vi "test - Round Trip -Array of Cluster of Enum and Array - Cluster.vi"(8 "error in (no error)":errorcluster, 11 "TestCase in":refnum<class "Python Data Tools Tests.lvclass">) -> (0 "error out":errorcluster, 3 "TestCase out":refnum<class "Python Data Tools Tests.lvclass">)   [LabVIEW 2013, in "Python Data Tools Tests.lvclass"]
uses:
  Python Data Tools Tests.lvclass
  <vilib>/addons/_JKI Toolkits/VI Tester/TestCase.llb/TestCase.lvclass
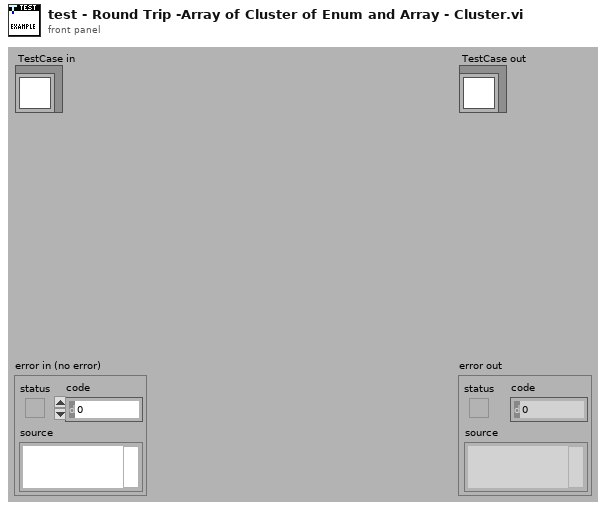
[diagram p1: front panel]
types:
  T1 = cluster{enum16{"Case1", "Case2", "AnotherCase"}, i32[]}[]
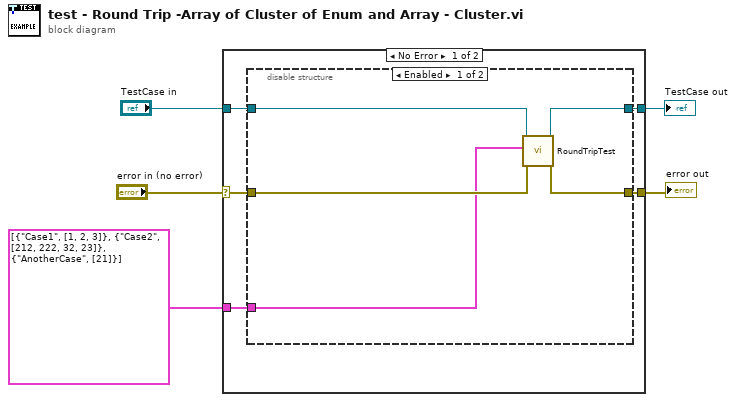
[diagram p0: block diagram]
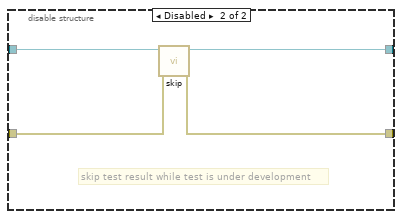
[diagram p2: hidden frame]
diagram:
  n1 = case shown="No Error" "error in (no error)" {
    selector: "error in (no error)" -> [w8 w21]
    tunnel: [w7 w21] -> w4
    tunnel: [w9 w20] -> w2
    tunnel: "TestCase in" -> [w10 w20]
    tunnel: T1 [{enum."Case1", [1, 2, 3]}, {enum."Case2", [212, 222, 32, 23]}, {enum."AnotherCase", [21]}] -> [w6 _]
    frame No Error {
      n2 = disable-structure shown="Enabled" {
        disable-tunnel: w10 -> [w15 w19]
        disable-tunnel: [w14 w16] -> w9
        disable-tunnel: w8 -> [w12 w18]
        disable-tunnel: [w13 w17] -> w7
        disable-tunnel: w6 -> [w11 _]
        frame Enabled {
          n3 = call "RoundTripTest.vi"("error in (no error)"=w12, "Variant"=w11, "TestCase in"=w15) -> ("error out"=w13:errorcluster, "TestCase out"=w14:refnum<class "Python Data Tools Tests.lvclass">)  [unwired: 6 in, 1 out]
        }
        frame Disabled {
          # "skip test result while test is under development"
          n4 = call <vilib>:"skip.vi"("error in (no error)"=w18, "TestCase in"=w19) -> ("error out"=w17:errorcluster, "TestCase out"=w16:refnum<class "Python Data Tools Tests.lvclass">)  [unwired: 8 in]
        }
      }
    }
    frame Error {
    }
  }
  "error out" <- w4
  "TestCase out" <- w2
